vi "Execute.OpenSequence.vi"(8 "error in (no error)":errorcluster, 11 "State Variables":T1={"NIVS.BaseLogPath"=path "", "NIVS.SystemDefinitionFile"=path "", "NIVS.Events"={"SequenceEvent"=refnum, "SystemChangeEvent"=refnum, "WorkspaceEvent"=refnum}, "NIVS.SequenceState"=enum."Idle", "NIVS.GatewayIPAddress"="", "NIVS.DataLogSpecRef"=refnum, "NIVS.DataLogManagerRef"=refnum, "NIVS.LogSessionGUID"="", "NIVS.WorkspaceManager"=refnum, "NIVS.Deployed"=FALSE, "NIVS.ProfileRef"=refnum, "NIVS.ProfileCallback"=refnum, "NIVS.SystemStateRefs"={"CustDatRef"=refnum, "EvtRef"=refnum}, "UI.Abort"=refnum, "UI.Pause"=refnum, "UI.EnableLogging"=refnum, "UI.Start"=refnum, "UI.LogChannels"=refnum, "UI.StartIteration"=refnum, "UI.StartStep"=refnum, "UI.Sequence"=refnum, "UI.PreviewMode"=refnum, "UI.Graph"=refnum, "UI.BaseFileName"=refnum, "UI.Profiles"=refnum, "UI.CurrentStep"=refnum, "UI.CurrentIteration"=refnum, "UI.TotalIterations"=refnum, "Sequence.AbortChannel"="", "Sequence.StepInfoChannel"="", "Sequence.Iterations"=0, "Sequence.IterationInfoChannel"="", "Sequence.#ofColumns"=0, "Events.State"=refnum, "Events.Test Result"=refnum, "Events.Progress"=refnum, "INI.Settings"={"Build Location"=path "C:/Simple Sequence Editor/SequenceRepo", "LoggingLocation"=path ""}, "UI.Skip"=refnum, "Sequence.SkipChannel"="", "Restart.Path"=path "", "UI.Duration"=refnum, "Sequence.DurationChannel"=""}) -> (0 "error out":errorcluster, 3 "State Variables":T1={"NIVS.BaseLogPath"=path "", "NIVS.SystemDefinitionFile"=path "", "NIVS.Events"={"SequenceEvent"=refnum, "SystemChangeEvent"=refnum, "WorkspaceEvent"=refnum}, "NIVS.SequenceState"=enum."Idle", "NIVS.GatewayIPAddress"="", "NIVS.DataLogSpecRef"=refnum, "NIVS.DataLogManagerRef"=refnum, "NIVS.LogSessionGUID"="", "NIVS.WorkspaceManager"=refnum, "NIVS.Deployed"=FALSE, "NIVS.ProfileRef"=refnum, "NIVS.ProfileCallback"=refnum, "NIVS.SystemStateRefs"={"CustDatRef"=refnum, "EvtRef"=refnum}, "UI.Abort"=refnum, "UI.Pause"=refnum, "UI.EnableLogging"=refnum, "UI.Start"=refnum, "UI.LogChannels"=refnum, "UI.StartIteration"=refnum, "UI.StartStep"=refnum, "UI.Sequence"=refnum, "UI.PreviewMode"=refnum, "UI.Graph"=refnum, "UI.BaseFileName"=refnum, "UI.Profiles"=refnum, "UI.CurrentStep"=refnum, "UI.CurrentIteration"=refnum, "UI.TotalIterations"=refnum, "Sequence.AbortChannel"="", "Sequence.StepInfoChannel"="", "Sequence.Iterations"=0, "Sequence.IterationInfoChannel"="", "Sequence.#ofColumns"=0, "Events.State"=refnum, "Events.Test Result"=refnum, "Events.Progress"=refnum, "INI.Settings"={"Build Location"=path "C:/Simple Sequence Editor/SequenceRepo", "LoggingLocation"=path ""}, "UI.Skip"=refnum, "Sequence.SkipChannel"="", "Restart.Path"=path "", "UI.Duration"=refnum, "Sequence.DurationChannel"=""})   [LabVIEW 2013, in "Simple Sequence Tools - Execution.lvlib"]
uses:
  Simple Sequence Tools - Execution.lvlib
  Types/Main.StateVariables.ctl
  Types/Execute.UserEventRefs.ctl
  <vilib>/NI Veristand/Execution/Workspace/SystemStateRegEventRef.ctl
  Types/Execution.SequenceState.ctl
  <vilib>/NI Veristand/Execution/DataLogging/DataLoggingSpecification Ref.ctl
  NationalInstruments.VeriStand.ClientAPI
  <vilib>/NI Veristand/Execution/DataLogging/IDataLogging Ref.ctl
  <vilib>/NI Veristand/Execution/Workspace/WorkspaceAPI.ctl
  NationalInstruments.VeriStand.RealTimeSequenceDefinitionApi
  <vilib>/NI Veristand/Execution/Workspace/SystemStateEventRef.ctl
  Shared/Types/INI.Settings
  Shared/SubVIs/Main.Constants.vi
  Shared/Simple Sequence Tools - Shared.lvlib
  <vilib>/NI Veristand/Execution/Workspace/NI_VS Workspace ExecutionAPI.lvlib
  <vilib>/NI Veristand/Execution/DataLogging/NI_VS Data Logging API.lvlib
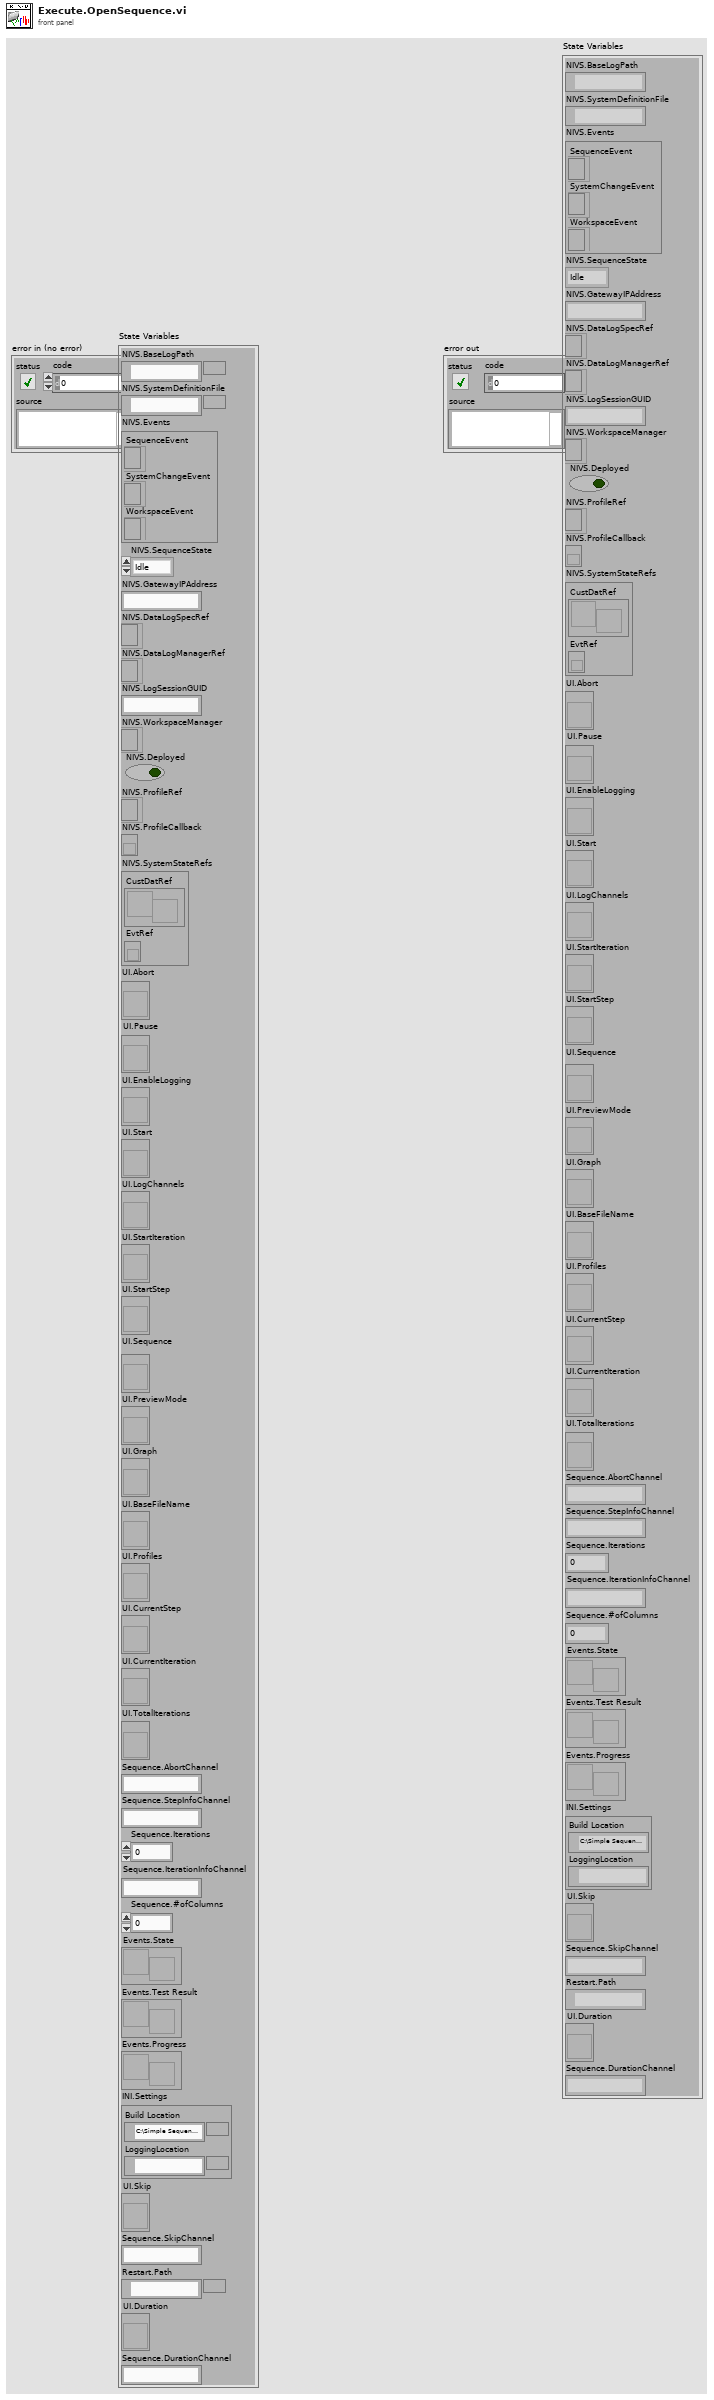
[diagram p1: front panel]
types:
  T1 = typedef "Simple Sequence Tools - Execution.lvlib/Main.StateVariables.ctl" = cluster{"NIVS.BaseLogPath":path, "NIVS.SystemDefinitionFile":path, "NIVS.Events":T2, "NIVS.SequenceState":T4, "NIVS.GatewayIPAddress":string, "NIVS.DataLogSpecRef":T5, "NIVS.DataLogManagerRef":T6, "NIVS.LogSessionGUID":string, "NIVS.WorkspaceManager":T7, "NIVS.Deployed":bool, "NIVS.ProfileRef":refnum<k24>, "NIVS.ProfileCallback":refnum<k27>, "NIVS.SystemStateRefs":T8, "UI.Abort":refnum<vi>, "UI.Pause":refnum<vi>, "UI.EnableLogging":refnum<vi>, "UI.Start":refnum<vi>, "UI.LogChannels":refnum<vi>, "UI.StartIteration":refnum<vi>, "UI.StartStep":refnum<vi>, "UI.Sequence":refnum<vi>, "UI.PreviewMode":refnum<vi>, "UI.Graph":refnum<vi>, "UI.BaseFileName":refnum<vi>, "UI.Profiles":refnum<vi>, "UI.CurrentStep":refnum<vi>, "UI.CurrentIteration":refnum<vi>, "UI.TotalIterations":refnum<vi>, "Sequence.AbortChannel":string, "Sequence.StepInfoChannel":string, "Sequence.Iterations":u32, "Sequence.IterationInfoChannel":string, "Sequence.#ofColumns":i32, "Events.State":refnum<user-event>, "Events.Test Result":refnum<user-event>, "Events.Progress":refnum<user-event>, "INI.Settings":T9, "UI.Skip":refnum<vi>, "Sequence.SkipChannel":string, "Restart.Path":path, "UI.Duration":refnum<vi>, "Sequence.DurationChannel":string}
  T2 = typedef "Simple Sequence Tools - Execution.lvlib/Execute.UserEventRefs.ctl" = cluster{"SequenceEvent":refnum<event-registration>, "SystemChangeEvent":T3, "WorkspaceEvent":refnum<event-registration>}
  T3 = typedef "NI_VS Workspace ExecutionAPI.lvlib/SystemStateRegEventRef.ctl" = refnum<event-registration>
  T4 = typedef "Simple Sequence Tools - Execution.lvlib/Execution.SequenceState.ctl" = enum16{"Idle", "Initializing", "Running", "Paused", "Finalizing", "Complete"}
  T5 = typedef "NI_VS Data Logging API.lvlib/DataLoggingSpecification Ref.ctl" = refnum<k24>
  T6 = typedef "NI_VS Data Logging API.lvlib/IDataLogging Ref.ctl" = refnum<k24>
  T7 = typedef "NI_VS Workspace ExecutionAPI.lvlib/WorkspaceAPI.ctl" = refnum<k24>
  T8 = typedef "NI_VS Workspace ExecutionAPI.lvlib/SystemStateEventRef.ctl" = cluster{"CustDatRef":refnum<user-event>, "EvtRef":refnum<k27>}
  T9 = typedef "Simple Sequence Tools - Shared.lvlib/INI.Settings" = cluster{"Build Location":path, "LoggingLocation":path}
  T10 = enum8{"Enabled", "Disabled", "Disabled and Grayed Out"}
  T11 = typedef "Simple Sequence Tools - Shared.lvlib/Saved.Sequence.ctl" = cluster{"Output Channels":T12[], "Item Names":string[][], "Step":T12, "Abort":T12, "Iterations":u32, "Iteration":T12, "Skip":T12, "Duration":T12}
  T12 = typedef "Simple Sequence Tools - Shared.lvlib/Channel.Properties.ctl" = cluster{"Name":string, "NodePath":string, "ScaleUnits":string}
  T13 = typedef "LVBoundsTypeDef.ctl" = cluster{"Width":u32, "Height":u32}
  T14 = typedef "Simple Sequence Tools - Execution.lvlib/Restart.Settings" = cluster{"LogFile":path, "Log Settings":T15[], "StimulusProfile":path, "StopIteration":u32, "StopStep":u32, "Log Channels":T19, "Base File Name":string, "Enable Logging":bool, "Profile":string, "StopDuration":dbl}
  T15 = typedef "NI_VS Data Logging API.lvlib/TDMS Channel Group.ctl" = cluster{"Group Name":string, "Group Description":string, "Group Properties":T16[], "Channels":T17[], "Time Channel Options":T18, "Time Channel Name":string}
  T16 = typedef "NI_VS Data Logging API.lvlib/TDMS Property.ctl" = cluster{"Name":string, "Value":variant}
  T17 = typedef "NI_VS Data Logging API.lvlib/TDMS Channel.ctl" = cluster{"Channel Name":string, "Channel Path":string, "Channel Description":string, "Channel Properties":T16[]}
  T18 = typedef "NI_VS Data Logging API.lvlib/Time Channel Options.ctl" = enum16{"No Time Channel", "Absolute Time", "System Time", "System Time - Microseconds", "Absolute Time as Double"}
  T19 = typedef "Simple Sequence Tools - Execution.lvlib/Log.SelectedChannels.ctl" = enum16{"Channels (No System Channel)", "Aliases", "All"}
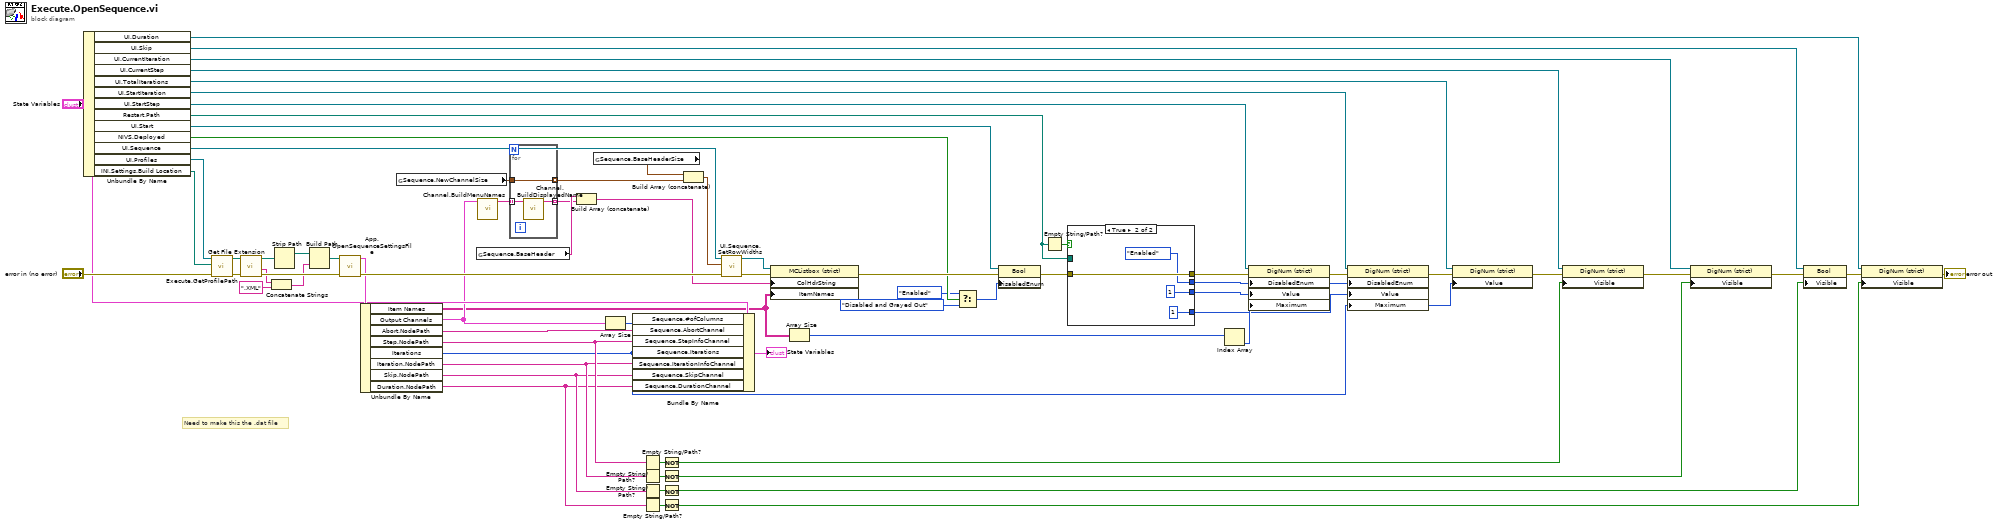
[diagram p0: block diagram]
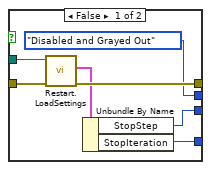
[diagram p2: hidden frame]
diagram:
  # "Need to make this the .dat file"
  n1 = Unbundle By Name("State Variables") -> ("UI.Duration"=w3:refnum<vi>, "UI.Skip"=w18:refnum<vi>, "UI.CurrentIteration"=w33:refnum<vi>, "UI.CurrentStep"=w34:refnum<vi>, "UI.TotalIterations"=w23:refnum<vi>, "UI.StartIteration"=w38:refnum<vi>, "UI.StartStep"=w28:refnum<vi>, "Restart.Path"=w11:path, "UI.Start"=w54:refnum<vi>, "NIVS.Deployed"=w52:bool, "UI.Sequence"=w62:refnum<vi>, "UI.Profiles"=w39:refnum<vi>, "INI.Settings.Build Location"=w20:path)
  n2 = call "Execute.GetProfilePath.vi"("error in (no error)"="error in (no error)", "base path"=w20, "Profiles"=w39) -> ("error out"=w46:errorcluster, "Path"=w48:path)  [unwired: 7 in]
  n3 = call <vilib>:"Get File Extension.vi"("error in (no error)"=w46, "file"=w48) -> ("error out"=w45:errorcluster, "filename without extension"=w43:string, "dup file"=w47:path)  [unwired: 6 in, 1 out]
  n4 = Concatenate Strings(w43, ".XML" ("string")) -> (w41:string)
  n5 = Strip Path(path=w47) -> (stripped path=w44:path)  [unwired: 1 out]
  n6 = Build Path(base path=w44, name or relative path=w41) -> (appended path=w40:path)
  n7 = call "App.OpenSequenceSettingsFile.vi"("error in (no error)"=w45, "selected path"=w40) -> ("error out"=w71:errorcluster, "Settings"=w60:T11)  [unwired: 8 in]
  n8 = Unbundle By Name(w60) -> ("Item Names"=w17:string[][], "Output Channels"=w55:T12[], "Abort.NodePath"=w58:string, "Step.NodePath"=w32:string, "Iterations"=w24:u32, "Iteration.NodePath"=w31:string, "Skip.NodePath"=w14:string, "Duration.NodePath"=w2:string)
  n9 = global read "Main.Constants.vi" "Sequence.NewChannelSize"() -> (w67:T13)
  n10 = global read "Main.Constants.vi" "Sequence.BaseHeader"() -> (w66:string[])
  n11 = call "Channel.BuildMenuNames.vi"("Aliases"=w55) -> ("Aliases Array"=w63:string[])  [unwired: 10 in]
  n12 = for {
    tunnel: w63 -> [w76] mode=indexing
    tunnel: [w75] -> w65 mode=indexing
    tunnel: [w74] -> w68 mode=indexing
    tunnel: w67 -> [w74]
    n13 = call "Channel.BuildDisplayedName.vi"("Path"=w76) -> ("Formated Path"=w75:string)  [unwired: 10 in]
  }
  n14 = Build Array (concatenate)(w66, w65) -> (w64:string[])
  n15 = global read "Main.Constants.vi" "Sequence.BaseHeaderSize"() -> (w69:T13[])
  n16 = Array Size(array=w55) -> (size(s)=w56:i32)
  n17 = Bundle By Name(cluster="State Variables", "Sequence.#ofColumns"=w56, "Sequence.AbortChannel"=w58, "Sequence.StepInfoChannel"=w32, "Sequence.Iterations"=w24, "Sequence.IterationInfoChannel"=w31, "Sequence.SkipChannel"=w14, "Sequence.DurationChannel"=w2) -> (→"State Variables":T1)
  n18 = Empty String/Path?(string/path=w32) -> (empty?=w29:bool)
  n19 = Empty String/Path?(string/path=w31) -> (empty?=w30:bool)
  n20 = Empty String/Path?(string/path=w14) -> (empty?=w16:bool)
  n21 = Empty String/Path?(string/path=w2) -> (empty?=w7:bool)
  n22 = Not(x=w29) -> (.not. x?=w22:bool)
  n23 = Not(x=w30) -> (.not. x?=w21:bool)
  n24 = Not(x=w16) -> (.not. x?=w15:bool)
  n25 = Not(x=w7) -> (.not. x?=w4:bool)
  n26 = Build Array (concatenate)(w69, w68) -> (w70:T13[])
  n27 = call "UI.Sequence.SetRowWidths.vi"("error in (no error)"=w71, "CellSize"=w70, "UI.SequenceRef"=w62) -> ("error out"=w72:errorcluster, "UI.SequenceRef"=w73:refnum<vi>)  [unwired: 7 in]
  n28 = property class="MCListbox (strict)"(reference=w73, error in=w72, "ColHdrString"=w64, "ItemNames"=w17) -> (error out=w53:errorcluster)  [unwired: 1 out]
  n29 = Array Size(array=w17) -> (size(s)=w37:i32[])
  n30 = Select(t=T10."Enabled" ("Disabled"), s=w52, f=T10."Disabled and Grayed Out" ("Disabled")) -> (s? t:f=w49:T10)
  n31 = property class="Bool"(reference=w54, error in=w53, "DisabledEnum"=w49) -> (error out=w13:errorcluster)  [unwired: 1 out]
  n32 = Empty String/Path?(string/path=w11) -> (empty?=w10:bool)
  n33 = case shown="True" w10 {
    tunnel: w13 -> [w83 w85]
    tunnel: [w82 w85] -> w12
    tunnel: w11 -> [w81 _]
    tunnel: [w78 u32 1 ("Value")] -> w9
    tunnel: [w79 u32 1 ("Value")] -> w8
    tunnel: [T10."Disabled and Grayed Out" ("Disabled") T10."Enabled" ("Disabled")] -> w1
    frame False {
      n34 = call "Restart.LoadSettings.vi"("error in"=w83, "path (use dialog)"=w81) -> ("error out"=w82:errorcluster, "Restart Settings"=w80:T14)  [unwired: 7 in, 1 out]
      n35 = Unbundle By Name(w80) -> ("StopStep"=w78:u32, "StopIteration"=w79:u32)
    }
    frame True {
    }
  }
  n36 = Index Array(array=w37) -> (element=w36:i32)  [unwired: 1 in]
  n37 = property class="DigNum (strict)"(reference=w28, error in=w12, "DisabledEnum"=w1, "Value"=w9, "Maximum"=w36) -> (error out=w27:errorcluster)  [unwired: 1 out]
  n38 = property class="DigNum (strict)"(reference=w38, error in=w27, "DisabledEnum"=w1, "Value"=w8, "Maximum"=w24) -> (error out=w26:errorcluster)  [unwired: 1 out]
  n39 = property class="DigNum (strict)"(reference=w23, error in=w26, "Value"=w24) -> (error out=w25:errorcluster)  [unwired: 1 out]
  n40 = property class="DigNum (strict)"(reference=w34, error in=w25, "Visible"=w22) -> (error out=w35:errorcluster)  [unwired: 1 out]
  n41 = property class="DigNum (strict)"(reference=w33, error in=w35, "Visible"=w21) -> (error out=w19:errorcluster)  [unwired: 1 out]
  n42 = property class="Bool"(reference=w18, error in=w19, "Visible"=w15) -> (error out=w6:errorcluster)  [unwired: 1 out]
  n43 = property class="DigNum (strict)"(reference=w3, error in=w6, "Visible"=w4) -> (error out=→"error out":errorcluster)  [unwired: 1 out]
